vi "Load Settings from XML.vi"(8 "error in (no error)":errorcluster, 11 "Settings in":T1={"Hardware Configuration"={"VISA resource name"="", "DAQ Type"=0, "Channel 1"={"Acquiring"=FALSE, "Enabled"=FALSE, "Terminal configuration"=0, "Range"=32767, "Coupling"=0}, "Channel 2"={"Acquiring"=FALSE, "Enabled"=FALSE, "Terminal configuration"=0, "Range"=0, "Coupling"=0}, "Timing"={"Sample Time [Time Units]"=0, "Actual Sample Time [s]"=0.0, "Samples per Iteration"=0, "Sample Clock Source"=0, "Time Units"=0, "t0"=timestamp(0 s since 1904-01-01)}, "PS Parameters"={"PS handle"=0, "PS Max_adc"=32767, "PS Enabled Array"=[], "PS Device Info"={"Driver Version"="", "USB Version"="", "Hardware"="", "Variant"="", "Batch and Serial"="", "Cal Date"="", "Kernel Version"="", "Digital HW Version"="", "Analogue HW Version"="", "Firmware 1"="", "Firmware 2"="", "MSO"=FALSE, "Number of Channels"=0}, "Channel 1 Buffer"=refnum, "Channel 2 Buffer"=refnum, "Resolution"=0, "USB Power"=FALSE}, "Trigger"={"Direction"=0, "Threshold [V]"=0.0, "Enabled"=FALSE, "Trigger Source"=0}, "Keithley Parameters"={"Previous End / Current Start"=0, "Quantity"=0}}, "Logging Configuration"={"Log File Base Path"=path "", "TDMS File Reference"=refnum, "Enabled"=FALSE, "Disk cache size"=0}} {"Hardware Configuration"."Keithley Parameters"."Quantity" items=["Current", "Voltage"]; "Hardware Configuration"."Trigger"."Trigger Source" items=["Channel 1"=0, "Channel 2"=1, "Ext."=4]; "Hardware Configuration"."Trigger"."Direction" items=["Falling", "Rising"]; "Hardware Configuration"."PS Parameters"."Resolution" items=["8", "12", "14", "15", "16"]; "Hardware Configuration"."Timing"."Time Units" items=["Seconds"]; "Hardware Configuration"."Timing"."Sample Clock Source" items=["Internal", "External"]; "Hardware Configuration"."Channel 2"."Coupling" items=["AC", "DC"]; "Hardware Configuration"."Channel 2"."Range" items=["0.01", "0.02", "0.05", "0.1", "0.2", "0.5", "1", "2", "5", "10", "20", "50", "100", "1000"]; "Hardware Configuration"."Channel 2"."Terminal configuration" items=["Referenced Single Ended", "Differential"]; "Hardware Configuration"."Channel 1"."Coupling" items=["AC", "DC"]; "Hardware Configuration"."Channel 1"."Range" items=["0.01", "0.02", "0.05", "0.1", "0.2", "0.5", "1", "2", "5", "10", "20", "50", "100", "1000"]; "Hardware Configuration"."Channel 1"."Terminal configuration" items=["Referenced Single Ended", "Differential"]; "Hardware Configuration"."DAQ Type" items=["Simulated", "Tektronics DPO2k/3k/4k", "PicoScope 2000a Series", "Keithley DMM7510", "PicoScope 5000a Series"]}) -> (0 "error out":errorcluster, 3 "Settings out":T1={"Hardware Configuration"={"VISA resource name"="", "DAQ Type"=0, "Channel 1"={"Acquiring"=FALSE, "Enabled"=FALSE, "Terminal configuration"=0, "Range"=32767, "Coupling"=0}, "Channel 2"={"Acquiring"=FALSE, "Enabled"=FALSE, "Terminal configuration"=0, "Range"=0, "Coupling"=0}, "Timing"={"Sample Time [Time Units]"=0, "Actual Sample Time [s]"=0.0, "Samples per Iteration"=0, "Sample Clock Source"=0, "Time Units"=0, "t0"=timestamp(0 s since 1904-01-01)}, "PS Parameters"={"PS handle"=0, "PS Max_adc"=32767, "PS Enabled Array"=[], "PS Device Info"={"Driver Version"="", "USB Version"="", "Hardware"="", "Variant"="", "Batch and Serial"="", "Cal Date"="", "Kernel Version"="", "Digital HW Version"="", "Analogue HW Version"="", "Firmware 1"="", "Firmware 2"="", "MSO"=FALSE, "Number of Channels"=0}, "Channel 1 Buffer"=refnum, "Channel 2 Buffer"=refnum, "Resolution"=0, "USB Power"=FALSE}, "Trigger"={"Direction"=0, "Threshold [V]"=0.0, "Enabled"=FALSE, "Trigger Source"=0}, "Keithley Parameters"={"Previous End / Current Start"=0, "Quantity"=0}}, "Logging Configuration"={"Log File Base Path"=path "", "TDMS File Reference"=refnum, "Enabled"=FALSE, "Disk cache size"=0}} {"Hardware Configuration"."Keithley Parameters"."Quantity" items=["Current", "Voltage"]; "Hardware Configuration"."Trigger"."Trigger Source" items=["Channel 1"=0, "Channel 2"=1, "Ext."=4]; "Hardware Configuration"."Trigger"."Direction" items=["Falling", "Rising"]; "Hardware Configuration"."PS Parameters"."Resolution" items=["8", "12", "14", "15", "16"]; "Hardware Configuration"."Timing"."Time Units" items=["Seconds"]; "Hardware Configuration"."Timing"."Sample Clock Source" items=["Internal", "External"]; "Hardware Configuration"."Channel 2"."Coupling" items=["AC", "DC"]; "Hardware Configuration"."Channel 2"."Range" items=["0.01", "0.02", "0.05", "0.1", "0.2", "0.5", "1", "2", "5", "10", "20", "50", "100", "1000"]; "Hardware Configuration"."Channel 2"."Terminal configuration" items=["Referenced Single Ended", "Differential"]; "Hardware Configuration"."Channel 1"."Coupling" items=["AC", "DC"]; "Hardware Configuration"."Channel 1"."Range" items=["0.01", "0.02", "0.05", "0.1", "0.2", "0.5", "1", "2", "5", "10", "20", "50", "100", "1000"]; "Hardware Configuration"."Channel 1"."Terminal configuration" items=["Referenced Single Ended", "Differential"]; "Hardware Configuration"."DAQ Type" items=["Simulated", "Tektronics DPO2k/3k/4k", "PicoScope 2000a Series", "Keithley DMM7510", "PicoScope 5000a Series"]})   [LabVIEW 2016, in "Settings.lvlib"]
doc: "Attempts to load previous user specified settings from an XML file.\n\nThis VI will not generate an error. If a suitable XML file can't be loaded and parsed then it will simply return the default settings."
uses:
  Settings.lvlib
  Settings.ctl
  Acquisition/Hardware Configuration.ctl
  Acquisition/Signal Type.ctl
  Terminal Configuration.ctl
  Range.ctl
  Coupling.ctl
  Sampling Clock Source.ctl
  Time Units.ctl
  Resolution.ctl
  Trigger Direction.ctl
  Trigger Source.ctl
  Quantity.ctl
  Logging/Logging Configuration.ctl
  <vilib>/Utility/xml.llb/Read From XML File(string).vi
  <vilib>/Utility/xml.llb/Write to XML File(string).vi
  Acquisition/Acquisition.lvlib
  Logging/Logging.lvlib
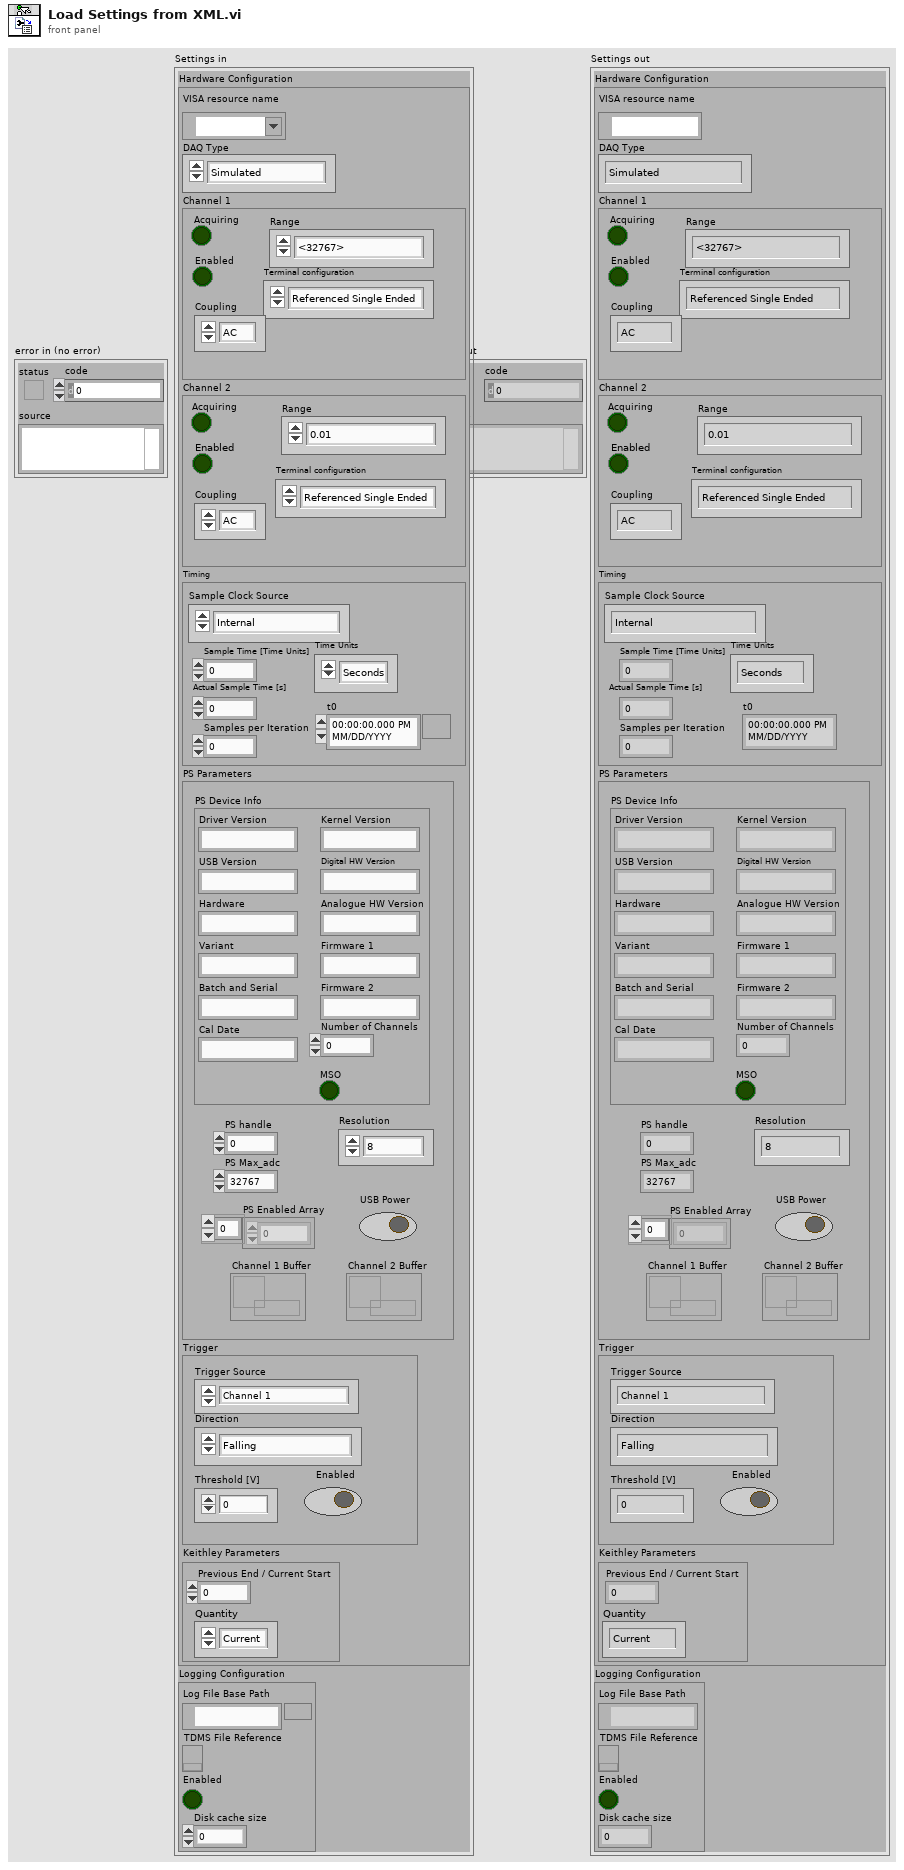
[diagram p1: front panel]
types:
  T1 = typedef "Settings.lvlib/Settings.ctl" = cluster{"Hardware Configuration":T2, "Logging Configuration":T13}
  T2 = typedef "Acquisition.lvlib/Hardware Configuration.ctl" = cluster{"VISA resource name":refnum<visa-resource-name>, "DAQ Type":T3, "Channel 1":cluster{"Acquiring":bool, "Enabled":bool, "Terminal configuration":T4, "Range":T5, "Coupling":T6}, "Channel 2":cluster{"Acquiring":bool, "Enabled":bool, "Terminal configuration":T4, "Range":T5, "Coupling":T6}, "Timing":cluster{"Sample Time [Time Units]":u32, "Actual Sample Time [s]":dbl, "Samples per Iteration":u32, "Sample Clock Source":T7, "Time Units":T8, "t0":timestamp}, "PS Parameters":cluster{"PS handle":i16, "PS Max_adc":i16, "PS Enabled Array":i16[], "PS Device Info":cluster{"Driver Version":string, "USB Version":string, "Hardware":string, "Variant":string, "Batch and Serial":string, "Cal Date":string, "Kernel Version":string, "Digital HW Version":string, "Analogue HW Version":string, "Firmware 1":string, "Firmware 2":string, "MSO":bool, "Number of Channels":i16}, "Channel 1 Buffer":refnum<data-value>, "Channel 2 Buffer":refnum<data-value>, "Resolution":T9, "USB Power":bool}, "Trigger":cluster{"Direction":T10, "Threshold [V]":dbl, "Enabled":bool, "Trigger Source":T11}, "Keithley Parameters":cluster{"Previous End / Current Start":i32, "Quantity":T12}}
  T3 = typedef "Acquisition.lvlib/Signal Type.ctl" = u16
  T4 = typedef "Settings.lvlib/Terminal Configuration.ctl" = u16
  T5 = typedef "Settings.lvlib/Range.ctl" = u16
  T6 = typedef "Settings.lvlib/Coupling.ctl" = i16
  T7 = typedef "Settings.lvlib/Sampling Clock Source.ctl" = u16
  T8 = typedef "Settings.lvlib/Time Units.ctl" = u32
  T9 = typedef "Settings.lvlib/Resolution.ctl" = i32
  T10 = typedef "Settings.lvlib/Trigger Direction.ctl" = u16
  T11 = typedef "Settings.lvlib/Trigger Source.ctl" = u16
  T12 = typedef "Settings.lvlib/Quantity.ctl" = u16
  T13 = typedef "Logging.lvlib/Logging Configuration.ctl" = cluster{"Log File Base Path":path, "TDMS File Reference":refnum<k34>, "Enabled":bool, "Disk cache size":u64}
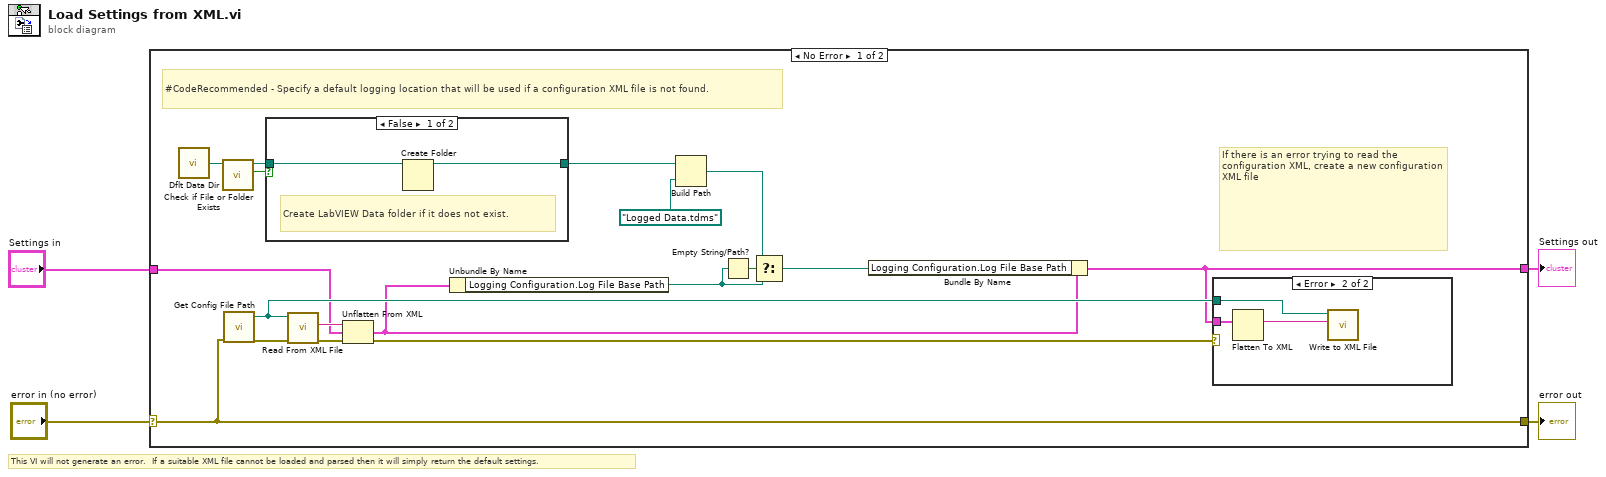
[diagram p0: block diagram]
diagram:
  # "This VI will not generate an error.  If a suitable XML file cannot be loaded and parsed then it will simply return the default settings."
  n1 = case shown="No Error" "error in (no error)" {
    selector: "error in (no error)" -> [w20 w30]
    tunnel: [w20 w30] -> w3
    tunnel: "Settings in" -> [w15 w29]
    tunnel: [w9 w29] -> w1
    frame No Error {
      # "If there is an error trying to read the configuration XML, create a new configuration XML file"
      # "#CodeRecommended - Specify a default logging location that will be used if a configuration XML file is not found."
      n2 = call <vilib>:"Dflt Data Dir.vi"() -> ("App:Default Data Directory"=w8:path)
      n3 = call <vilib>:"Check if File or Folder Exists.vi"("path"=w8) -> ("file or folder exists?"=w7:bool, "dup path"=w6:path)  [unwired: 8 in, 1 out]
      n4 = call "Get Config File Path.vi"("error in (no error)"=w20) -> ("error out"=w22:errorcluster, "XML File Path"=w18:path)  [unwired: 9 in]
      n5 = case shown="False" w7 {
        tunnel: w6 -> [w24 w25]
        tunnel: [w23 w25] -> w5
        frame False {
          # "Create LabVIEW Data folder if it does not exist."
          n6 = Create Folder(path (use dialog)=w24) -> (created path=w23:path)  [unwired: 2 in, 2 out]
        }
        frame True {
        }
      }
      n7 = call-poly <vilib>:"Read From XML File.vi"("error in (no error)"=w22, "XML File Path"=w18) -> ("error out"=w17:errorcluster, "XML Elements"=w21:string)  [unwired: 7 in, 1 out]
      n8 = Unflatten From XML(xml string=w21, type=w15, error in (no error)=w17) -> (value=w11:T1, error out=w16:errorcluster)
      n9 = Unbundle By Name(w11) -> ("Logging Configuration.Log File Base Path"=w13:path)
      n10 = Build Path(base path=w5, name or relative path=path "Logged Data.tdms" ("App:Default Data Directory")) -> (appended path=w12:path)
      n11 = Empty String/Path?(string/path=w13) -> (empty?=w14:bool)
      n12 = Select(t=w12, s=w14, f=w13) -> (s? t:f=w10:path)
      n13 = Bundle By Name(cluster=w11, "Logging Configuration.Log File Base Path"=w10) -> (w9:T1)
      n14 = case shown="Error" w16 {
        tunnel: w9 -> [_ w28]
        tunnel: w18 -> [_ w26]
        frame No Error {
        }
        frame Error {
          n15 = Flatten To XML(anything=w28) -> (xml string=w27:string)
          n16 = call-poly <vilib>:"Write to XML File.vi"("XML Input"=w27, "XML File Path"=w26) -> ()  [unwired: 7 in, 3 out]
        }
      }
    }
    frame Error {
    }
  }
  "error out" <- w3
  "Settings out" <- w1
